vi "Register Descriptors.vi"(8 "error in (no error)":errorcluster, 11 "gRPC ID":T1) -> (0 "error out":errorcluster, 3 "gRPC ID Out":T1)   [LabVIEW 2019, in "MicronGRPCGeneratedServer.lvlib"]
uses:
  MicronGRPCGeneratedServer.lvlib
  <vilib>/gRPC/LabVIEW gRPC Library/Shared/grpcId.ctl
  <vilib>/gRPC/LabVIEW gRPC Library/grpc-lvsupport-release.lvlib
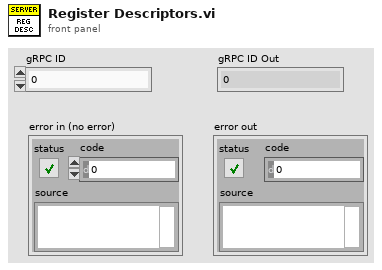
[diagram p1: front panel]
types:
  T1 = typedef "grpc-lvsupport-release.lvlib/grpcId.ctl" = u64
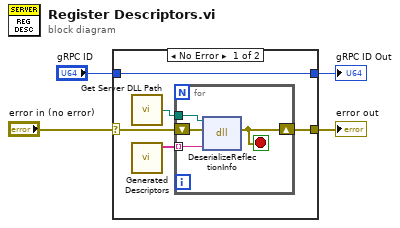
[diagram p0: block diagram]
diagram:
  n1 = case shown="No Error" "error in (no error)" {
    selector: "error in (no error)" -> [w7 w15]
    tunnel: [w5 w14] -> w1
    tunnel: [w6 w15] -> w4
    tunnel: "gRPC ID" -> [w5 w14]
    frame No Error {
      n2 = call <vilib>:"Get Server DLL Path.vi"() -> ("server dll path"=w9:path)
      n3 = call "Generated Descriptors.vi"() -> ("Descriptor Strings"=w8:string[])  [unwired: 11 in]
      n4 = for {
        tunnel: w9 -> [w13]
        tunnel: w8 -> [w12] mode=indexing
        shift-right: [w10] -> w6
        shift-left: w7 -> [w11]
        stop <- w10 stop-if-true
        n5 = dll-call lib="?" fn="DeserializeReflectionInfo"(path in=w13, error in=w11, "serializedDescriptor"=w12) -> (error out=w10:errorcluster)  [unwired: 3 in, 1 out]
      }
    }
    frame Error {
    }
  }
  "error out" <- w4
  "gRPC ID Out" <- w1
